vi "Get Hotkey.vi"(8 "error in (no error)":errorcluster, 11 "File Path":path) -> (0 "error out":errorcluster, 3 "Hotkey Values":T1)   [LabVIEW 2020, in "MacroAssert.lvlib"]
doc: "Gets all hotkey combinations from a config file."
uses:
  MacroAssert.lvlib
  CTLs/Hotkey Values.ctl
  CTLs/Hotkey Type.ctl
  fad5b3ff-ec19-4c01-b830-00555cb39235.vi
  <vilib>/Utility/config.llb/Read Key (String).vi
  <vilib>/Utility/error.llb/Error Cluster From Error Code.vi
  <vilib>/ErrorRing/Error Ring.xnode
  <vilib>/Utility/config.llb/NI_LVConfig.lvlib
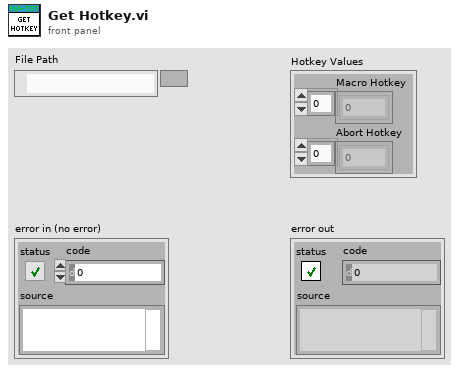
[diagram p1: front panel]
types:
  T1 = typedef "MacroAssert.lvlib/Hotkey Values.ctl" = cluster{"Macro Hotkey":enum16{"0", "1", "2", "3", "4", "5", "6", "7", "8", "9", "A", "B", "C", "D", "E", "F", "G", "H", "I", "J", "K", "L", "M", "N", "O", "P", "Q", "R", "S", "T", "U", "V", "W", "X", "Y", "Z", "F1", "F2", "F3", "F4", "F5", "F6", "F7", "F8", "F9", "F10", "F11", "F12", "F13", "F14", "F15", "ADD", "BACK", "BACKSLASH", "CAPITAL", "COMMA", "DECIMAL", "DELETE", "DIVIDE", "DOWN", "END", "EQUALS", "ESCAPE", "GRAVE (`)", "HOME", "INSERT", "LBRACKET", "LCONTROL", "LEFT", "L ALT", "LSHIFT", "LWIN", "MINUS", "MULTIPLY", "NEXT", "NUMLOCK", "NUMPAD_0", "NUMPAD_1", "NUMPAD_2", "NUMPAD_3", "NUMPAD_4", "NUMPAD_5", "NUMPAD_6", "NUMPAD_7", "NUMPAD_8", "NUMPAD_9", "PAUSE", "PERIOD", "PRIOR (PG UP)", "RBRACKET", "RCONTROL", "RETURN", "RIGHT", "R ALT", "RSHIFT", "RWIN", "SCROLL", "SEMICOLON", "SLASH", "SPACE", "SUBTRACT", "TAB", "UP", "ENTER (num pad)", "' (quote)"}[], "Abort Hotkey":enum16{"0", "1", "2", "3", "4", "5", "6", "7", "8", "9", "A", "B", "C", "D", "E", "F", "G", "H", "I", "J", "K", "L", "M", "N", "O", "P", "Q", "R", "S", "T", "U", "V", "W", "X", "Y", "Z", "F1", "F2", "F3", "F4", "F5", "F6", "F7", "F8", "F9", "F10", "F11", "F12", "F13", "F14", "F15", "ADD", "BACK", "BACKSLASH", "CAPITAL", "COMMA", "DECIMAL", "DELETE", "DIVIDE", "DOWN", "END", "EQUALS", "ESCAPE", "GRAVE (`)", "HOME", "INSERT", "LBRACKET", "LCONTROL", "LEFT", "L ALT", "LSHIFT", "LWIN", "MINUS", "MULTIPLY", "NEXT", "NUMLOCK", "NUMPAD_0", "NUMPAD_1", "NUMPAD_2", "NUMPAD_3", "NUMPAD_4", "NUMPAD_5", "NUMPAD_6", "NUMPAD_7", "NUMPAD_8", "NUMPAD_9", "PAUSE", "PERIOD", "PRIOR (PG UP)", "RBRACKET", "RCONTROL", "RETURN", "RIGHT", "R ALT", "RSHIFT", "RWIN", "SCROLL", "SEMICOLON", "SLASH", "SPACE", "SUBTRACT", "TAB", "UP", "ENTER (num pad)", "' (quote)"}[]}
  T2 = typedef "MacroAssert.lvlib/Hotkey Type.ctl" = enum16{"Macro Hotkey", "Abort Hotkey"}
  T3 = typedef "NI_LVConfig.lvlib/Config Data RefNum.ctl" = refnum<k1>
  T4 = enum16{"0", "1", "2", "3", "4", "5", "6", "7", "8", "9", "A", "B", "C", "D", "E", "F", "G", "H", "I", "J", "K", "L", "M", "N", "O", "P", "Q", "R", "S", "T", "U", "V", "W", "X", "Y", "Z", "F1", "F2", "F3", "F4", "F5", "F6", "F7", "F8", "F9", "F10", "F11", "F12", "F13", "F14", "F15", "ADD", "BACK", "BACKSLASH", "CAPITAL", "COMMA", "DECIMAL", "DELETE", "DIVIDE", "DOWN", "END", "EQUALS", "ESCAPE", "GRAVE (`)", "HOME", "INSERT", "LBRACKET", "LCONTROL", "LEFT", "L ALT", "LSHIFT", "LWIN", "MINUS", "MULTIPLY", "NEXT", "NUMLOCK", "NUMPAD_0", "NUMPAD_1", "NUMPAD_2", "NUMPAD_3", "NUMPAD_4", "NUMPAD_5", "NUMPAD_6", "NUMPAD_7", "NUMPAD_8", "NUMPAD_9", "PAUSE", "PERIOD", "PRIOR (PG UP)", "RBRACKET", "RCONTROL", "RETURN", "RIGHT", "R ALT", "RSHIFT", "RWIN", "SCROLL", "SEMICOLON", "SLASH", "SPACE", "SUBTRACT", "TAB", "UP", "ENTER (num pad)", "' (quote)"}
  T5 = enum16{"0", "1", "2", "3", "4", "5", "6", "7", "8", "9", "A", "B", "C", "D", "E", "F", "G", "H", "I", "J", "K", "L", "M", "N", "O", "P", "Q", "R", "S", "T", "U", "V", "W", "X", "Y", "Z", "F1", "F2", "F3", "F4", "F5", "F6", "F7", "F8", "F9", "F10", "F11", "F12", "F13", "F14", "F15", "ADD", "BACK", "BACKSLASH", "CAPITAL", "COMMA", "DECIMAL", "DELETE", "DIVIDE", "DOWN", "END", "EQUALS", "ESCAPE", "GRAVE (`)", "HOME", "INSERT", "LBRACKET", "LCONTROL", "LEFT", "L ALT", "LSHIFT", "LWIN", "MINUS", "MULTIPLY", "NEXT", "NUMLOCK", "NUMPAD_0", "NUMPAD_1", "NUMPAD_2", "NUMPAD_3", "NUMPAD_4", "NUMPAD_5", "NUMPAD_6", "NUMPAD_7", "NUMPAD_8", "NUMPAD_9", "PAUSE", "PERIOD", "PRIOR (PG UP)", "RBRACKET", "RCONTROL", "RETURN", "RIGHT", "R ALT", "RSHIFT", "RWIN", "SCROLL", "SEMICOLON", "SLASH", "SPACE", "SUBTRACT", "TAB", "UP", "ENTER (num pad)", "' (quote)"}[]
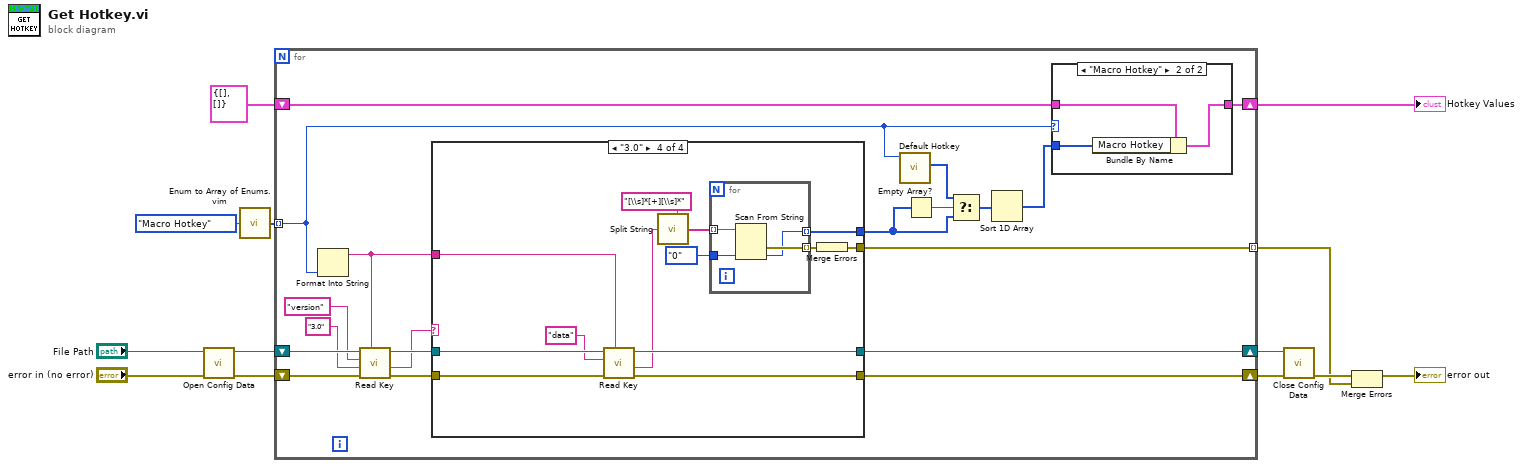
[diagram p0: block diagram]
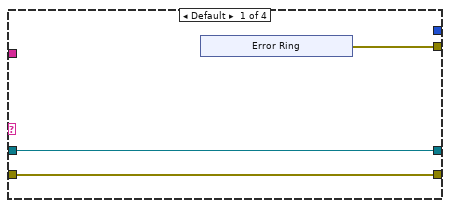
[diagram p2: hidden frame]
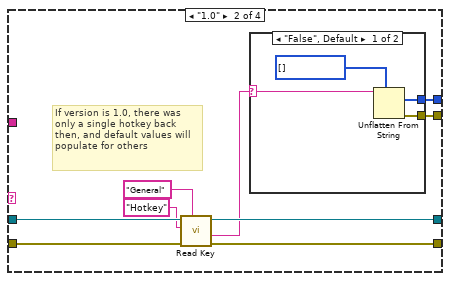
[diagram p3: hidden frame]
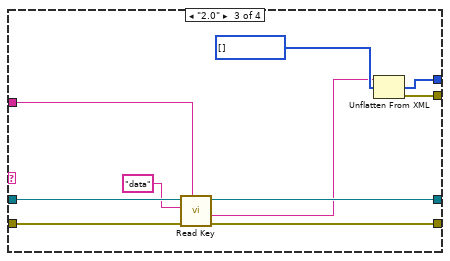
[diagram p5: hidden frame]
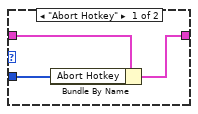
[diagram p6: hidden frame]
diagram:
  n1 = call <vilib>:"Open Config Data.vi"("error in (no error)"="error in (no error)", "configuration file path"="File Path") -> ("error out"=w12:errorcluster, "refnum"=w13:T3)  [unwired: 7 in, 1 out]
  n2 = call "Enum to Array of Enums.vim"("enum"=Hotkey_Type."Macro Hotkey" ("Hotkey Type")) -> ("array of enums"=w8:T2[])
  n3 = for {
    shift-right: [w20] -> w10
    shift-left: w13 -> [w29]
    shift-right: [w22] -> w11
    shift-left: w12 -> [w32]
    tunnel: [w21] -> w5 mode=indexing
    tunnel: w8 -> [w16] mode=indexing
    shift-right: [w30] -> w3
    shift-left: T1 {"Macro Hotkey"=[], "Abort Hotkey"=[]} -> [w31]
    n4 = Format Into String(w16) -> (resulting string=w23:string)  [unwired: 3 in, 1 out]
    n5 = call-poly <vilib>:"Read Key.vi"("section"=w23, "error in (no error)"=w32, "default value"="3.0", "key"="version", "refnum"=w29) -> ("error out"=w26:errorcluster, "value"=w24:string, "refnum out"=w25:T3)  [unwired: 3 in, 1 out]
    n6 = case shown="\"3.0\"" w24 {
      tunnel: w25 -> [w35 w49 w63 w75]
      tunnel: [w33 w43 w62 w66] -> w21
      tunnel: [_ w48 w61 w65] -> w18
      tunnel: [w35 w47 w60 w76] -> w20
      tunnel: w26 -> [w34 w46 w59 w74]
      tunnel: [w34 w45 w58 w67] -> w22
      tunnel: w23 -> [_ _ w56 w73]
      frame Default {
        n7 = xnode "Error Ring"() -> ("error out"=w33:errorcluster)
      }
      frame "1.0" {
        # "If version is 1.0, there was only a single hotkey back then, and default values will populate for others"
        n8 = call-poly <vilib>:"Read Key.vi"("section"="General", "error in (no error)"=w46, "key"="Hotkey", "refnum"=w49) -> ("error out"=w45:errorcluster, "value"=w42:string, "refnum out"=w47:T3)  [unwired: 4 in, 1 out]
        n9 = case shown="\"False\", Default" w42 {
          selector: w42 -> [w50 _]
          tunnel: [w53 _] -> w48
          tunnel: [w52 _] -> w43
          frame "False", Default {
            w51 = T5 [] items=["0", "1", "2", "3", "4", "5", "6", "7", "8", "9", "A", "B", "C", "D", "E", "F", "G", "H", "I", "J", "K", "L", "M", "N", "O", "P", "Q", "R", "S", "T", "U", "V", "W", "X", "Y", "Z", "F1", "F2", "F3", "F4", "F5", "F6", "F7", "F8", "F9", "F10", "F11", "F12", "F13", "F14", "F15", "ADD", "BACK", "BACKSLASH", "CAPITAL", "COMMA", "DECIMAL", "DELETE", "DIVIDE", "DOWN", "END", "EQUALS", "ESCAPE", "GRAVE (`)", "HOME", "INSERT", "LBRACKET", "LCONTROL", "LEFT", "L ALT", "LSHIFT", "LWIN", "MINUS", "MULTIPLY", "NEXT", "NUMLOCK", "NUMPAD_0", "NUMPAD_1", "NUMPAD_2", "NUMPAD_3", "NUMPAD_4", "NUMPAD_5", "NUMPAD_6", "NUMPAD_7", "NUMPAD_8", "NUMPAD_9", "PAUSE", "PERIOD", "PRIOR (PG UP)", "RBRACKET", "RCONTROL", "RETURN", "RIGHT", "R ALT", "RSHIFT", "RWIN", "SCROLL", "SEMICOLON", "SLASH", "SPACE", "SUBTRACT", "TAB", "UP", "ENTER (num pad)", "' (quote)"] ("Hotkey out")
            n10 = Unflatten From String(type=w51, binary string=w50) -> (value=w53:T5, error out=w52:errorcluster)  [unwired: 3 in, 1 out]
          }
          frame "" {
          }
        }
      }
      frame "2.0" {
        w57 = T5 [] items=["0", "1", "2", "3", "4", "5", "6", "7", "8", "9", "A", "B", "C", "D", "E", "F", "G", "H", "I", "J", "K", "L", "M", "N", "O", "P", "Q", "R", "S", "T", "U", "V", "W", "X", "Y", "Z", "F1", "F2", "F3", "F4", "F5", "F6", "F7", "F8", "F9", "F10", "F11", "F12", "F13", "F14", "F15", "ADD", "BACK", "BACKSLASH", "CAPITAL", "COMMA", "DECIMAL", "DELETE", "DIVIDE", "DOWN", "END", "EQUALS", "ESCAPE", "GRAVE (`)", "HOME", "INSERT", "LBRACKET", "LCONTROL", "LEFT", "L ALT", "LSHIFT", "LWIN", "MINUS", "MULTIPLY", "NEXT", "NUMLOCK", "NUMPAD_0", "NUMPAD_1", "NUMPAD_2", "NUMPAD_3", "NUMPAD_4", "NUMPAD_5", "NUMPAD_6", "NUMPAD_7", "NUMPAD_8", "NUMPAD_9", "PAUSE", "PERIOD", "PRIOR (PG UP)", "RBRACKET", "RCONTROL", "RETURN", "RIGHT", "R ALT", "RSHIFT", "RWIN", "SCROLL", "SEMICOLON", "SLASH", "SPACE", "SUBTRACT", "TAB", "UP", "ENTER (num pad)", "' (quote)"] ("Hotkey out")
        n11 = call-poly <vilib>:"Read Key.vi"("section"=w56, "error in (no error)"=w59, "key"="data", "refnum"=w63) -> ("error out"=w58:errorcluster, "value"=w55:string, "refnum out"=w60:T3)  [unwired: 4 in, 1 out]
        n12 = Unflatten From XML(xml string=w55, type=w57) -> (value=w61:T5, error out=w62:errorcluster)  [unwired: 1 in]
      }
      frame "3.0" {
        n13 = call-poly <vilib>:"Read Key.vi"("section"=w73, "error in (no error)"=w74, "key"="data", "refnum"=w75) -> ("error out"=w67:errorcluster, "value"=w64:string, "refnum out"=w76:T3)  [unwired: 4 in, 1 out]
        n14 = call <vilib>:"Split String.vi"("Split Pattern"="[\\s]*[+][\\s]*", "Input String"=w64) -> ("Split String"=w70:string[])  [unwired: 5 in]
        n15 = for {
          tunnel: w70 -> [w80] mode=indexing
          tunnel: T4."0" ("keyType 3") -> [w79]
          tunnel: [w77] -> w65 mode=indexing
          tunnel: [w78] -> w71 mode=indexing
          n16 = Scan From String(input string=w80, default 1=w79) -> (error out=w78:errorcluster, output 1=w77:T4)  [unwired: 3 in, 2 out]
        }
        n17 = Merge Errors(w71) -> (w66:errorcluster)
      }
    }
    n18 = call "Default Hotkey.vi"("Hotkey Type"=w16) -> ("Hotkey"=w17:T5)  [unwired: 9 in, 1 out]
    n19 = Empty Array?(array=w18) -> (empty?=w19:bool)
    n20 = Select(t=w17, s=w19, f=w18) -> (s? t:f=w15:T5)
    n21 = Sort 1D Array(array=w15) -> (sorted array=w14:T5)
    n22 = case shown="\"Macro Hotkey\"" w16 {
      tunnel: w31 -> [w83 w86]
      tunnel: [w82 w85] -> w30
      tunnel: w14 -> [w81 w84]
      frame "Abort Hotkey" {
        n23 = Bundle By Name(cluster=w83, "Abort Hotkey"=w81) -> (w82:T1)
      }
      frame "Macro Hotkey" {
        n24 = Bundle By Name(cluster=w86, "Macro Hotkey"=w84) -> (w85:T1)
      }
    }
  }
  "Hotkey Values" <- w3
  n25 = call <vilib>:"Close Config Data.vi"("error in (no error)"=w11, "refnum"=w10) -> ("error out"=w6:errorcluster)  [unwired: 8 in, 1 out]
  n26 = Merge Errors(w6, w5) -> (→"error out":errorcluster)
